vi "Lighting Test Software 4.vi"() -> ()   [LabVIEW 2020]
panel:
  in  "Tab Control":enum32{"Map", "Settings"}(tab)
  in  "Slide":dbl(slide)=0.7342857142857143 scale=0.0..1.0
  in  "Array 3":cluster{"Color Box":u32, "Slide":dbl}[][](array[cluster])=[[{"Color Box"=12303291, "Slide"=10.0}, {"Color Box"=12303291, "Slide"=10.0}, {"Color Box"=12303291, "Slide"=10.0}, {"Color Box"=12303291, "Slide"=10.0}, {"Color Box"=12303291, "Slide"=10.0}, {"Color Box"=12303291, "Slide"=10.0}], [{"Color Box"=12303291, "Slide"=10.0}, {"Color Box"=12303291, "Slide"=10.0}, {"Color Box"=12303291, "Slide"=10.0}, {"Color Box"=12303291, "Slide"=10.0}, {"Color Box"=12303291, "Slide"=10.0}, {"Color Box"=12303291, "Slide"=10.0}], [{"Color Box"=12303291, "Slide"=10.0}, {"Color Box"=12303291, "Slide"=10.0}, {"Color Box"=12303291, "Slide"=10.0}, {"Color Box"=12303291, "Slide"=10.0}, {"Color Box"=12303291, "Slide"=10.0}, {"Color Box"=12303291, "Slide"=10.0}], [{"Color Box"=12303291, "Slide"=10.0}, {"Color Box"=12303291, "Slide"=10.0}, {"Color Box"=12303291, "Slide"=10.0}, {"Color Box"=12303291, "Slide"=10.0}, {"Color Box"=0, "Slide"=0.0}, {"Color Box"=0, "Slide"=0.0}], [{"Color Box"=12303291, "Slide"=10.0}, {"Color Box"=12303291, "Slide"=10.0}, {"Color Box"=0, "Slide"=0.0}, {"Color Box"=12303291, "Slide"=10.0}, {"Color Box"=0, "Slide"=0.0}, {"Color Box"=0, "Slide"=0.0}], [{"Color Box"=0, "Slide"=0.0}, {"Color Box"=0, "Slide"=0.0}, {"Color Box"=12303291, "Slide"=10.0}, {"Color Box"=0, "Slide"=0.0}, {"Color Box"=0, "Slide"=0.0}, {"Color Box"=0, "Slide"=0.0}]] {"Slide" min=0.0 max=10.0 scale=-1.0..11.0 scale format="%_1g"}
  in  "Save Config":bool
  in  "Load Config":bool
  in  "Index":cluster{"Numeric":i32}[][](array[cluster])=[[{"Numeric"=3}, {"Numeric"=9}, {"Numeric"=2}, {"Numeric"=8}, {"Numeric"=19}, {"Numeric"=23}], [{"Numeric"=1}, {"Numeric"=11}, {"Numeric"=0}, {"Numeric"=10}, {"Numeric"=17}, {"Numeric"=21}], [{"Numeric"=5}, {"Numeric"=13}, {"Numeric"=4}, {"Numeric"=14}, {"Numeric"=27}, {"Numeric"=25}], [{"Numeric"=7}, {"Numeric"=15}, {"Numeric"=6}, {"Numeric"=12}, {"Numeric"=26}, {"Numeric"=24}], [{"Numeric"=29}, {"Numeric"=31}, {"Numeric"=-1}, {"Numeric"=18}, {"Numeric"=-1}, {"Numeric"=22}], [{"Numeric"=30}, {"Numeric"=-1}, {"Numeric"=16}, {"Numeric"=-1}, {"Numeric"=-1}, {"Numeric"=-1}]]
  in  "physical channels":refnum<k21>="Dev0/Ao0:15"
  in  "physical channels 2":refnum<k21>="Dev1/Ao0:15"
  out "error out":errorcluster
  out "specific error cleared?":bool
  in  "OK":bool
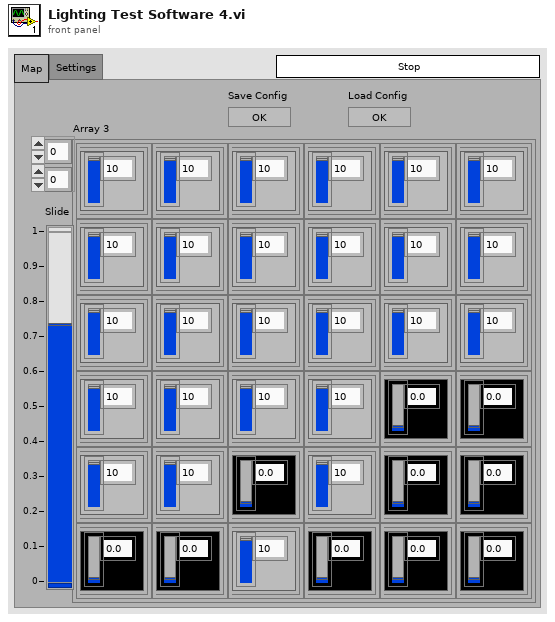
[diagram p1: front panel]
types:
  T1 = enum32{"invalid app kind", "Development System", "Run Time System", "Student Edition", "Embedded LabVIEW", "Evaluation", "Custom"}
  T2 = enum32{"Invalid", "Standard", "Closed", "Hidden", "Minimized", "Maximized"}
  T3 = cluster{"Core":cluster{"Current VI Reference":refnum<vi>, "Close Panel on Exit?":bool}, "Your Boolean data":bool}
  T4 = cluster{"Current VI Reference":refnum<vi>, "Close Panel on Exit?":bool}
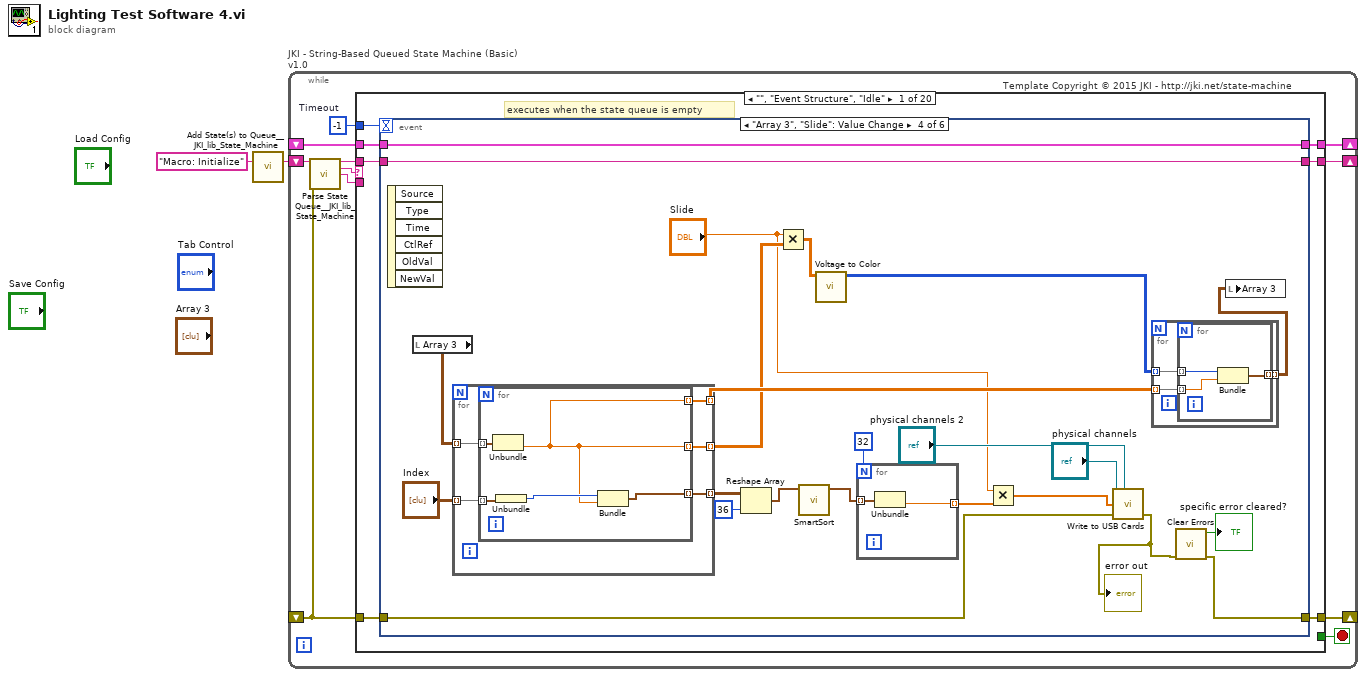
[diagram p0: block diagram]
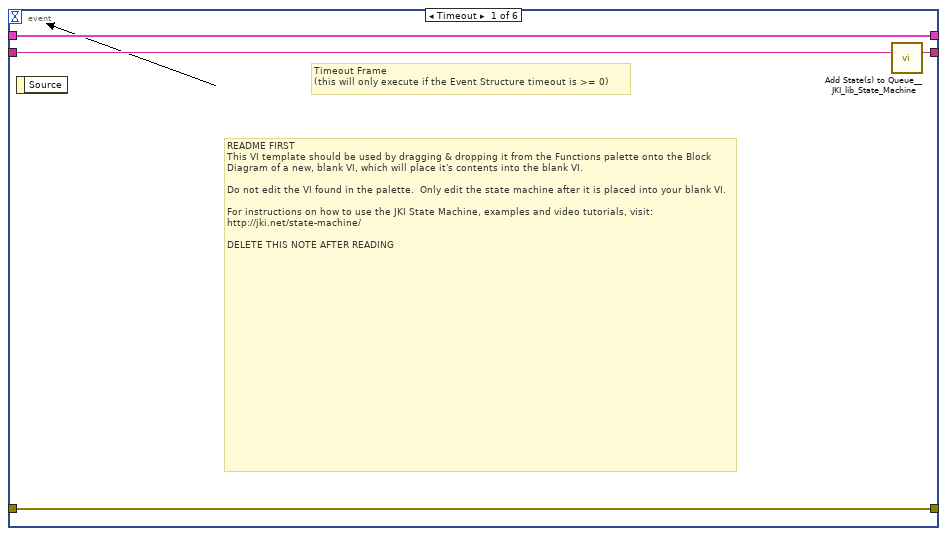
[diagram p2: hidden frame]
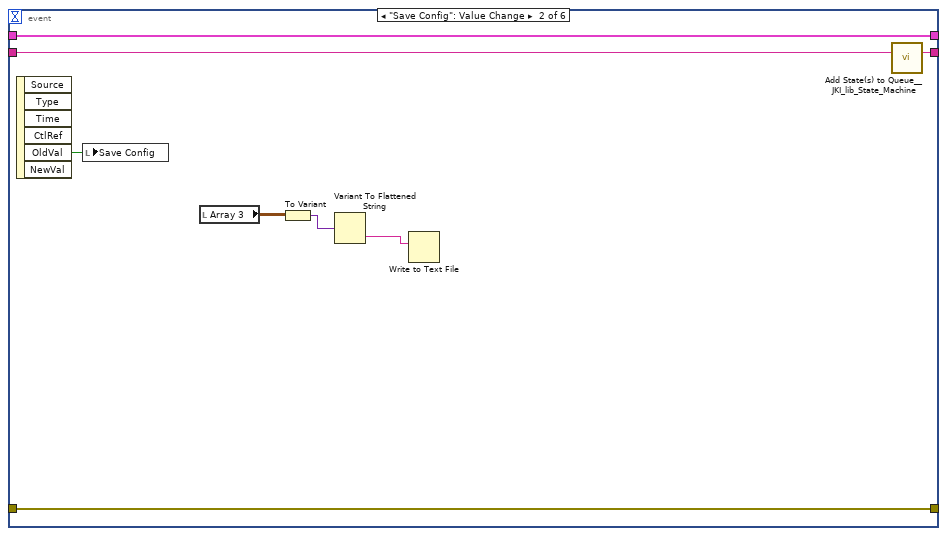
[diagram p3: hidden frame]
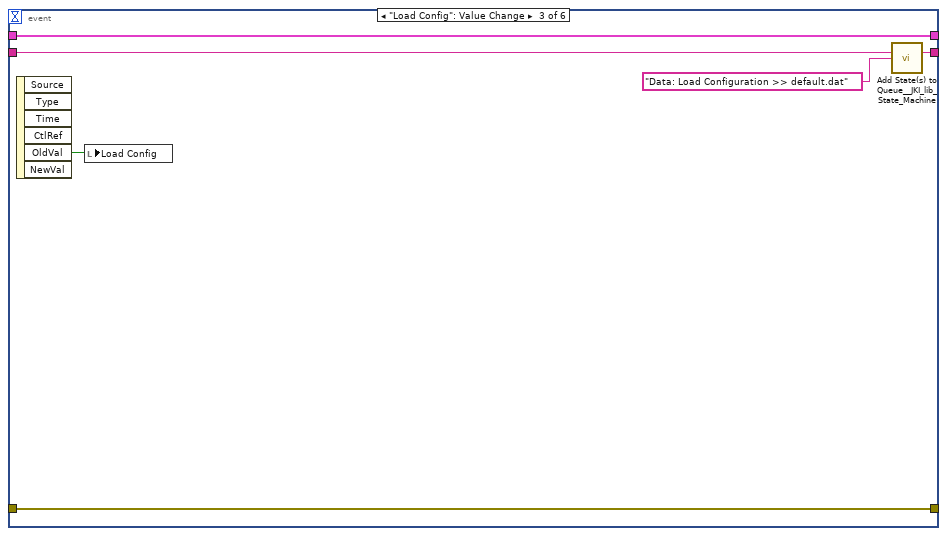
[diagram p4: hidden frame]
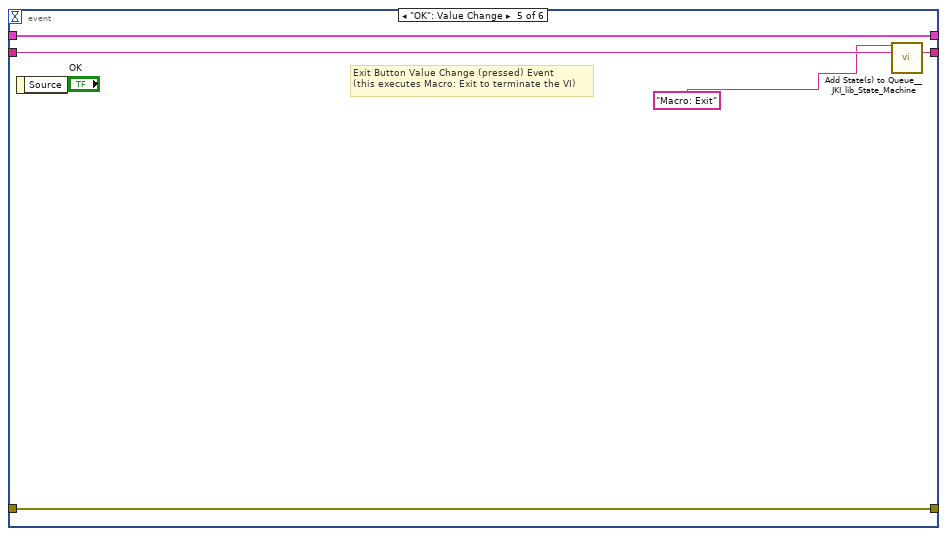
[diagram p5: hidden frame]
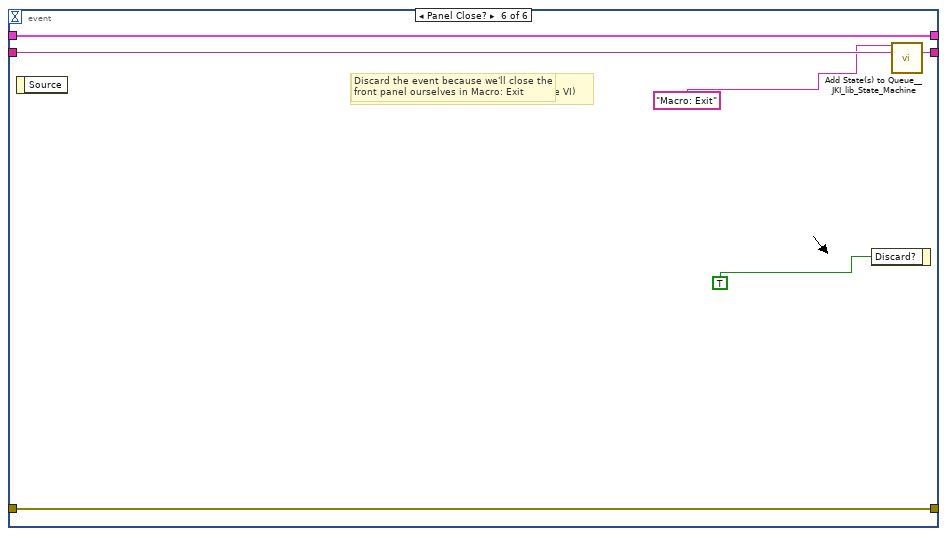
[diagram p6: hidden frame]
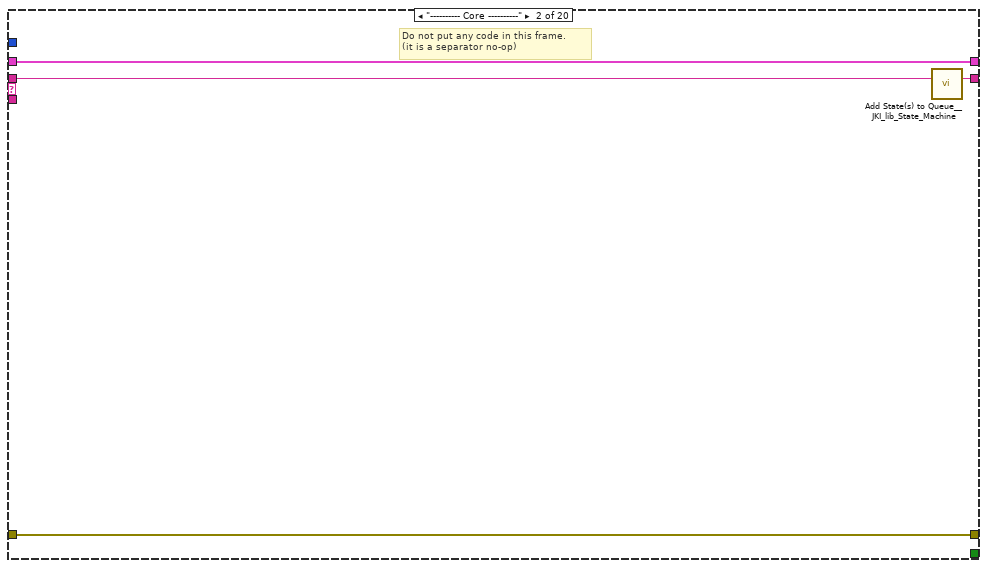
[diagram p7: hidden frame]
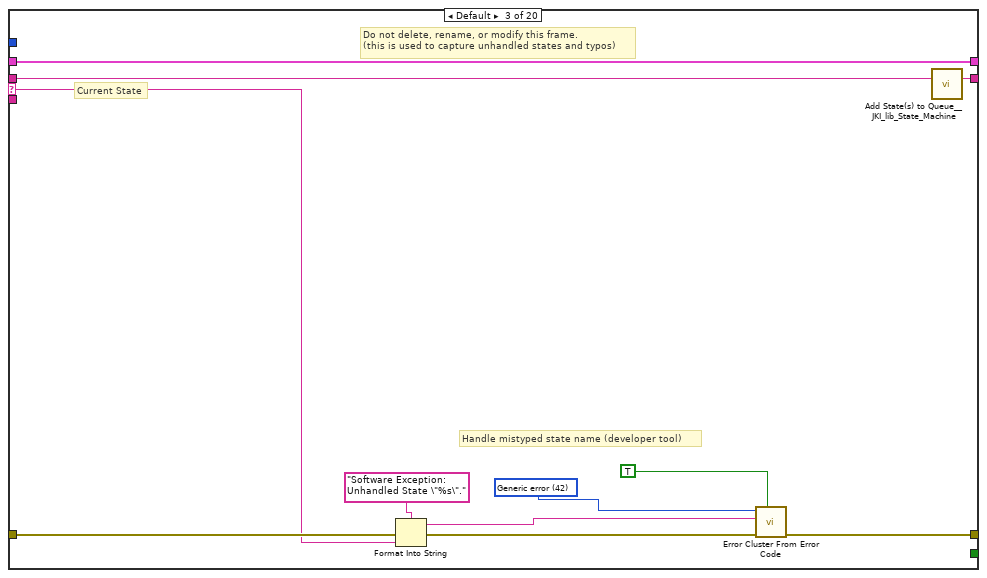
[diagram p8: hidden frame]
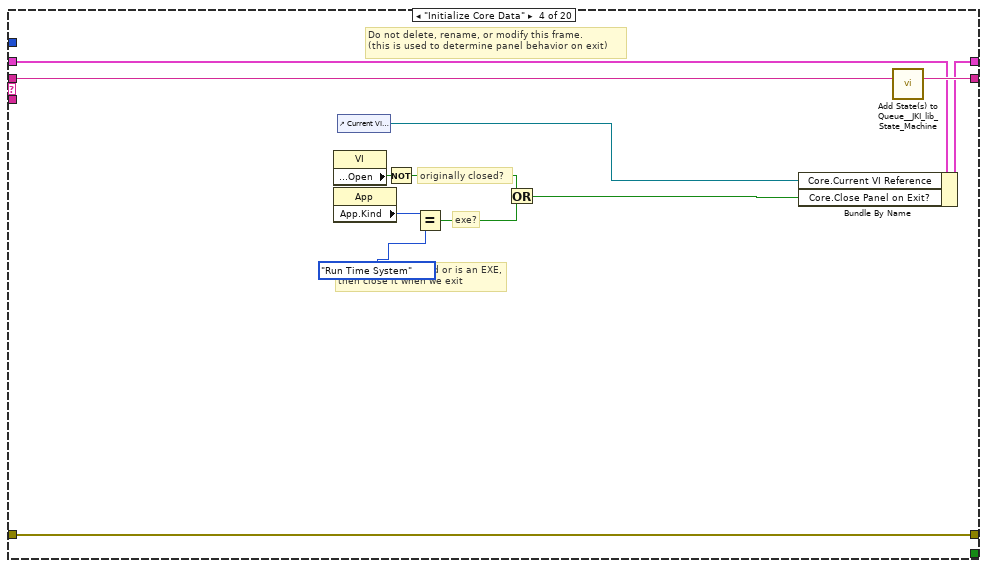
[diagram p9: hidden frame]
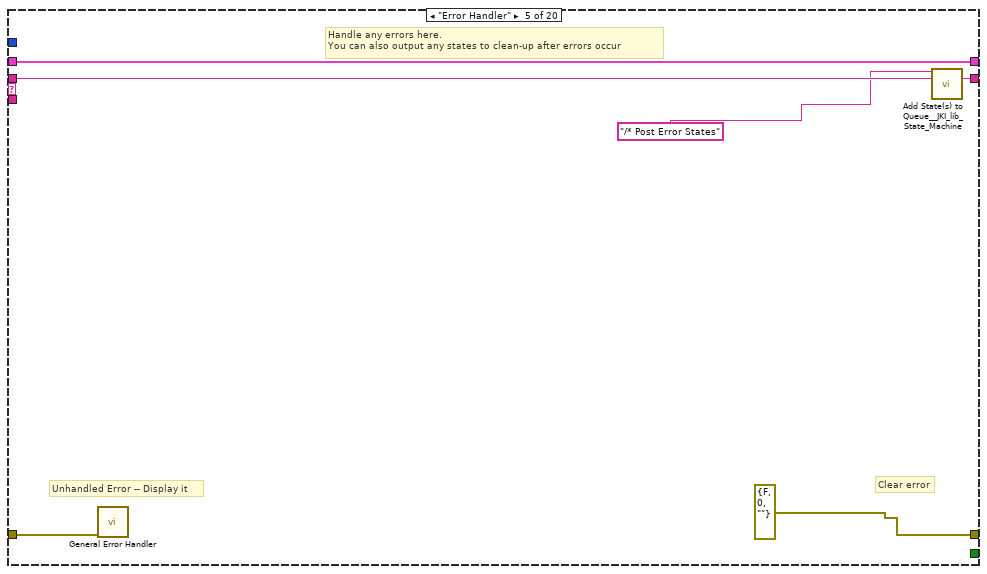
[diagram p10: hidden frame]
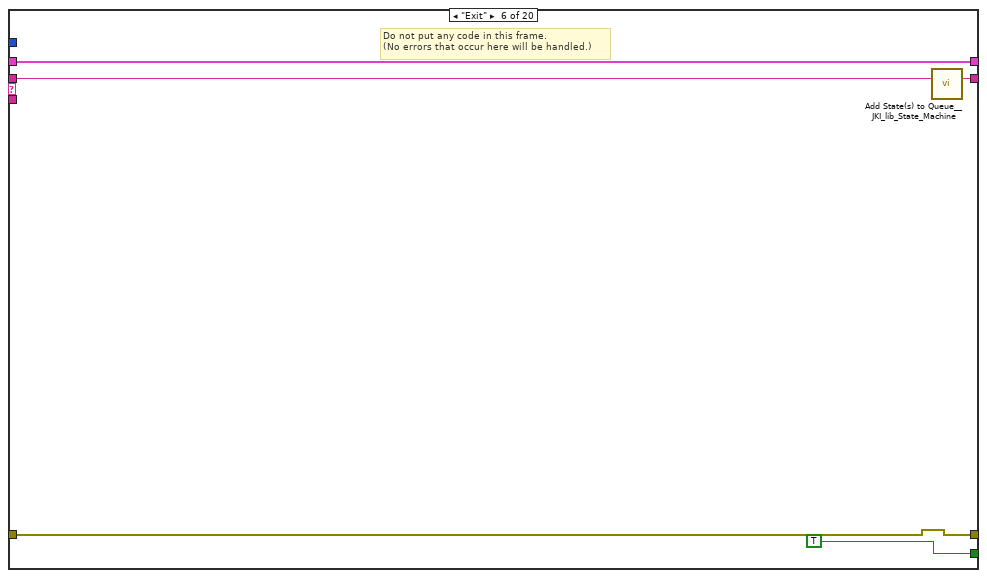
[diagram p11: hidden frame]
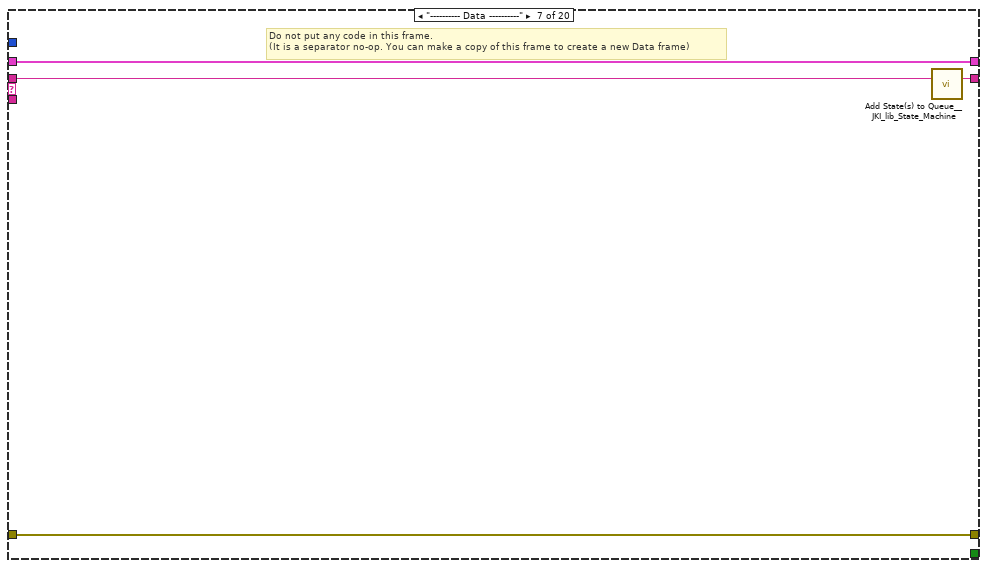
[diagram p12: hidden frame]
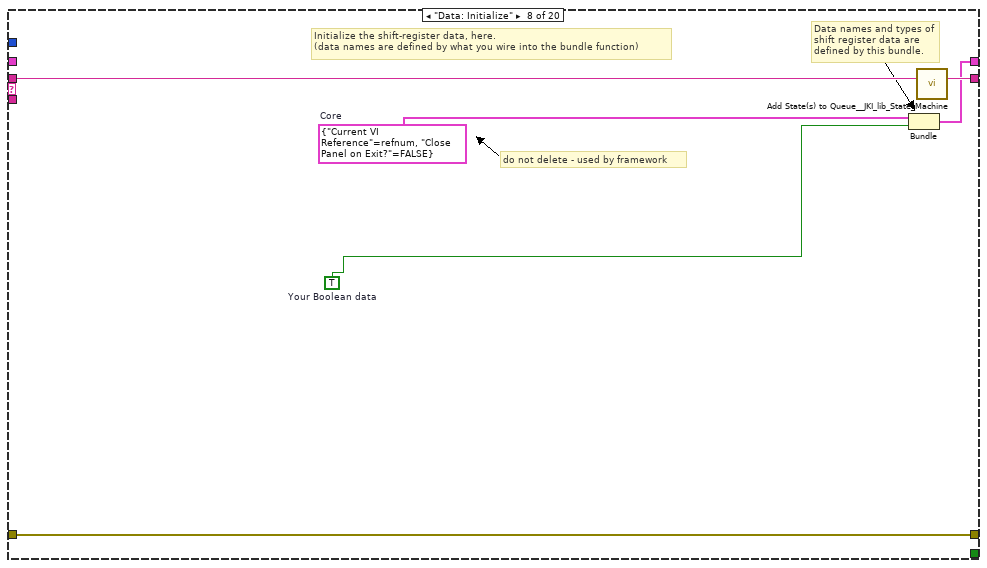
[diagram p13: hidden frame]
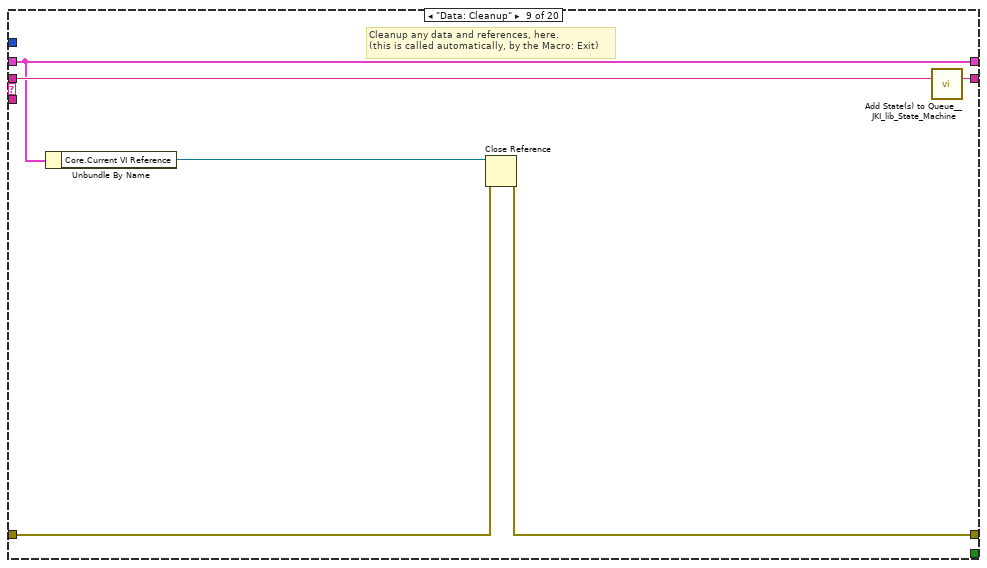
[diagram p14: hidden frame]
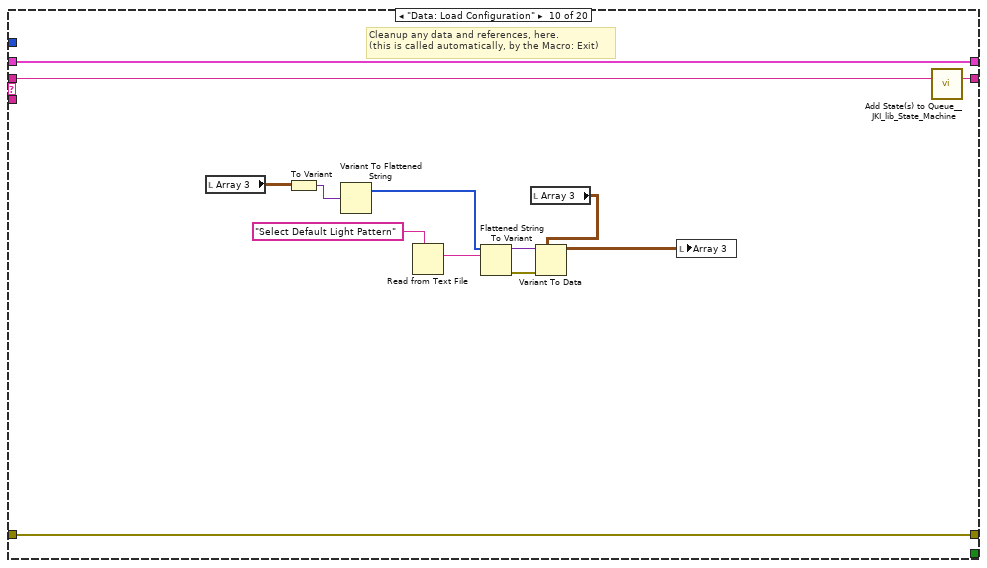
[diagram p15: hidden frame]
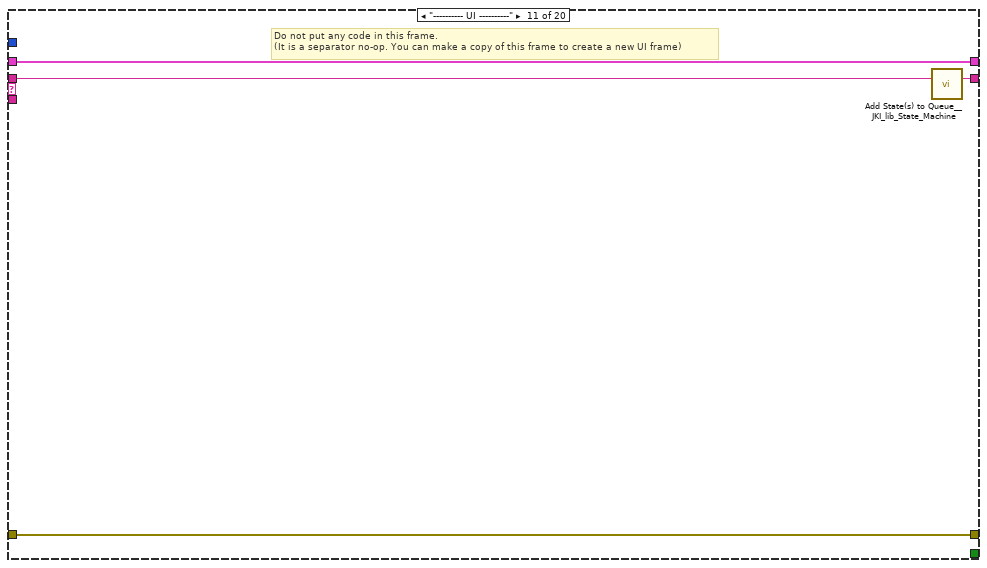
[diagram p16: hidden frame]
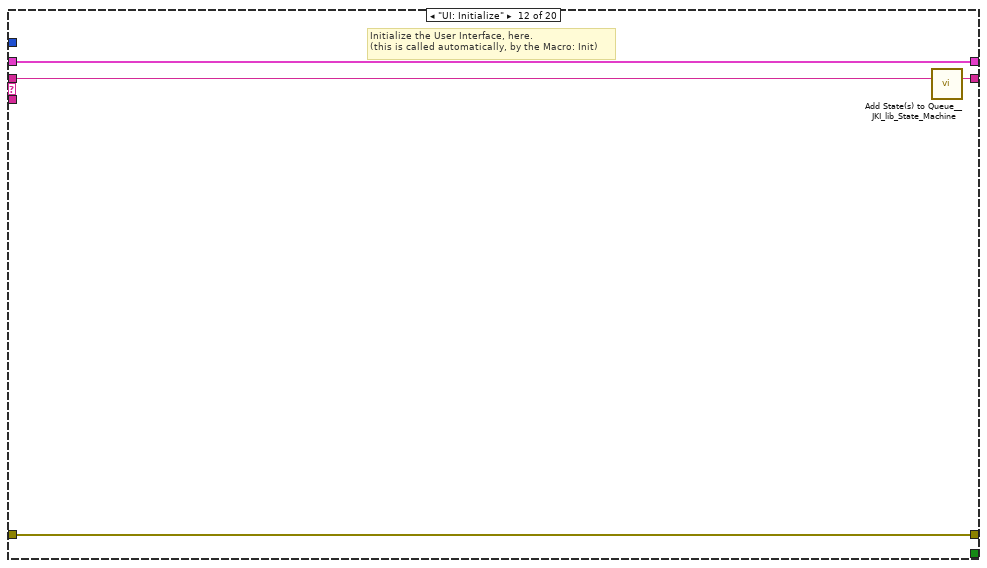
[diagram p17: hidden frame]
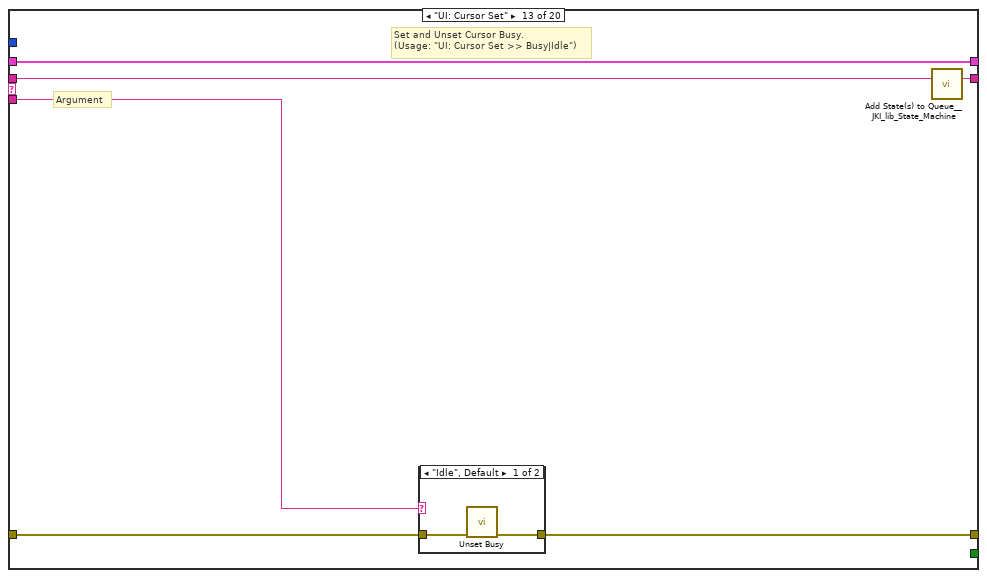
[diagram p18: hidden frame]
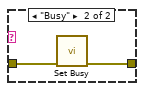
[diagram p19: hidden frame]
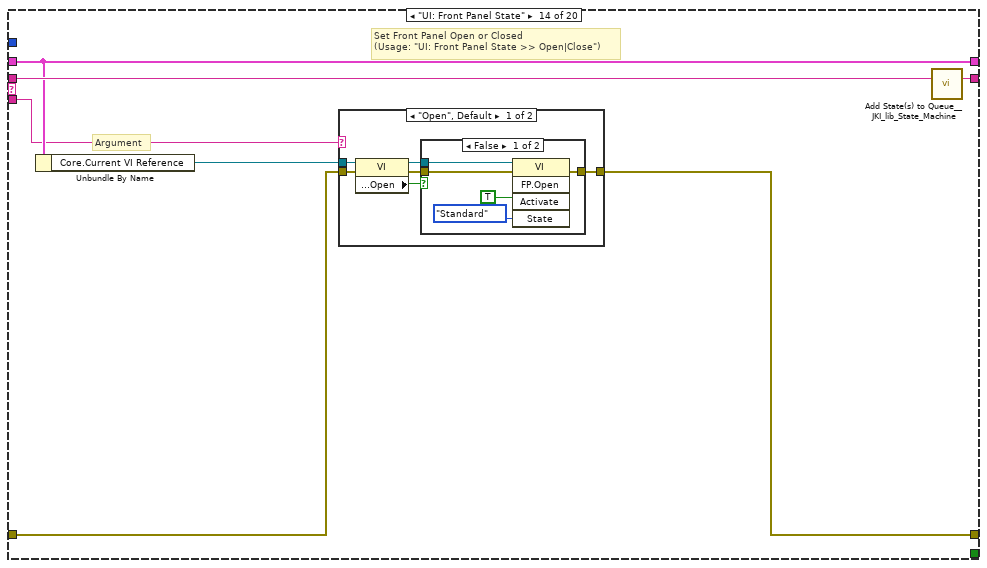
[diagram p20: hidden frame]
diagram:
  n1 = call <vilib>:"Add State(s) to Queue__JKI_lib_State_Machine.vi"("State(s) in (\"\")"="Macro: Initialize") -> ("States Out"=w2:string)  [unwired: 14 in]
  n2 = while "JKI - String-Based Queued State Machine (Basic) v1.0" {
    shift-right: [w6] -> _
    shift-left: _ -> [w5]
    shift-right: [w9] -> _
    shift-left: _ -> [w3]
    shift-right: [w8] -> _
    shift-left: w2 -> [w10]
    stop <- w7 stop-if-true
    w4 = -1  # Timeout
    # "Template Copyright © 2015 JKI - http://jki.net/state-machine"
    n3 = call <vilib>:"Parse State Queue__JKI_lib_State_Machine.vi"("State Queue"=w10, "Error In (no error)"=w3) -> ("Remaining States"=w12:string, "Current State"=w13:string, "Arguments"=w11:string)  [unwired: 11 in]
    n4 = case shown="\"\", \"Event Structure\", \"Idle\"" w13 {
      selector: w13 -> [_ _ w95 _ _ _ _ _ _ _ _ _ _ _ _ _ _ _ _ _]
      tunnel: w12 -> [w20 w94 w99 w117 w123 w128 w132 w138 w144 w157 w161 w165 w171 w182 w208 w213 w223 w227 w231 w235]
      tunnel: w11 -> [_ _ _ _ _ _ _ _ _ _ _ _ w166 w176 _ _ _ _ _ _]
      tunnel: w5 -> [w18 w91 w97 w108 w120 w125 w129 _ w139 w155 w158 w163 w169 w178 w205 w210 w220 w224 w228 w232]
      tunnel: [w17 w92 w101 w114 errorcluster {"status"=FALSE, "code"=0, "source"=""} ("error out") w124 w130 w133 w140 w154 w159 w162 w167 w179 w206 w211 w221 w225 w229 w233] -> w9
      tunnel: w3 -> [w16 w92 w100 w114 w119 w124 w130 w133 w141 w154 w159 w162 w168 w180 w206 w211 w221 w225 w229 w233]
      tunnel: [w19 w93 w98 w116 w122 w127 w131 w137 w143 w156 w160 w164 w170 w181 w207 w212 w222 w226 w230 w234] -> w8
      tunnel: [_ _ _ _ _ TRUE _ _ _ _ _ _ _ _ _ _ _ _ _ _] -> w7
      tunnel: [w15 w91 w97 w115 w120 w125 w129 w136 w139 w155 w158 w163 w169 w178 w205 w210 w220 w224 w228 w232] -> w6
      tunnel: w4 -> [w14 _ _ _ _ _ _ _ _ _ _ _ _ _ _ _ _ _ _ _]
      frame "", "Event Structure", "Idle" {
        # "executes when the state queue is empty"
        n5 = event shown="[3] \"Array 3\", \"Slide\": Value Change" {
          selector: _ -> [_ _ _ _ _ _]
          dyn-events: _ -> [_ _ _ _ _ _]
          timeout: w14 -> [_ _ _ _ _ _]
          tunnel: w20 -> [w24 w32 w38 w60 w84 w90]
          tunnel: [w23 w31 w37 w60 w83 w89] -> w19
          tunnel: w18 -> [w21 w29 w35 w61 w81 w87]
          tunnel: [w22 w30 w36 w46 w82 w88] -> w17
          tunnel: w16 -> [w22 w30 w36 w47 w82 w88]
          tunnel: [w21 w29 w35 w61 w81 w87] -> w15
          event Timeout {
            # "README FIRST\nThis VI template should be used by dragging & dropping it from the Functions palette onto the Block Diagram of a new, blank VI, which will place it's contents into the blank VI.\n\nDo not edit the VI found in the palette.  Only edit the state machine after it is placed into your blank VI.\n\nFor instructions on how to use the JKI State Machine, examples and video tutorials, visit:\nhttp://jki.net/state-machine/\n\nDELETE THIS NOTE AFTER READING"
            # "Timeout Frame\n(this will only execute if the Event Structure timeout is >= 0)"
            n6 = event-data() -> ()  [unwired: 1 in, 1 out]
            n7 = call <vilib>:"Add State(s) to Queue__JKI_lib_State_Machine.vi"("State(s) in (\"\")"=w24) -> ("States Out"=w23:string)  [unwired: 14 in]
          }
          event "Save Config": Value Change {
            n8 = event-data() -> ("OldVal"=w25:bool)  [unwired: 1 in, 5 out]
            n9 = local write "Save Config"(w25) -> ()
            n10 = local read "Array 3"() -> (w28:cluster{"Color Box":u32, "Slide":dbl}[][])
            n11 = To Variant(anything=w28) -> (Variant=w27:variant)
            n12 = Variant To Flattened String(Variant=w27) -> (data string=w26:string)  [unwired: 1 out]
            n13 = Write to Text File(text=w26) -> ()  [unwired: 3 in, 3 out]
            n14 = call <vilib>:"Add State(s) to Queue__JKI_lib_State_Machine.vi"("State(s) in (\"\")"=w32) -> ("States Out"=w31:string)  [unwired: 14 in]
          }
          event "Load Config": Value Change {
            n15 = event-data() -> ("OldVal"=w34:bool)  [unwired: 1 in, 5 out]
            n16 = local write "Load Config"(w34) -> ()
            n17 = call <vilib>:"Add State(s) to Queue__JKI_lib_State_Machine.vi"("State(s) in (\"\")"=w38, "State(s) at Back (\"\")"="Data: Load Configuration >> default.dat") -> ("States Out"=w37:string)  [unwired: 13 in]
          }
          event "Array 3", "Slide": Value Change {
            n18 = event-data() -> ()  [unwired: 1 in, 6 out]
            n19 = local read "Array 3"() -> (w59:cluster{"Color Box":u32, "Slide":dbl}[][])
            n20 = for {
              tunnel: w59 -> [w74] mode=indexing
              tunnel: [w73] -> w43 mode=indexing
              tunnel: [w72] -> w56 mode=indexing
              tunnel: "Index" -> [w71] mode=indexing
              tunnel: [w70] -> w54 mode=indexing
              n21 = for {
                tunnel: w74 -> [w79] mode=indexing
                tunnel: [w76] -> w73 mode=indexing
                tunnel: [w76] -> w72 mode=indexing
                tunnel: w71 -> [w78] mode=indexing
                tunnel: [w75] -> w70 mode=indexing
                n22 = Unbundle(w79) -> ("Slide"=w76:dbl)  [unwired: 1 out]
                n23 = Unbundle(w78) -> ("Numeric"=w77:i32)
                n24 = Bundle("Numeric"=w77, "Slide"=w76) -> (w75:cluster{"Numeric":i32, "Slide":dbl})  [unwired: 1 in]
              }
            }
            n25 = Reshape Array(w54, 36 ("dimension size")) -> (w52:cluster{"Numeric":i32, "Slide":dbl}[])
            n26 = Multiply(x="Slide", y=w43) -> (x*y=w42:dbl[][])
            n27 = call "SmartSort.vi"("Array in"=w52) -> ("Array out"=w51:cluster{"Numeric":i32, "Slide":dbl}[])  [unwired: 10 in]
            n28 = call "Voltage to Color.vi"("Array in"=w42) -> ("Array out"=w57:u32[][])  [unwired: 10 in]
            n29 = for {
              N: 32 -> [_]
              tunnel: w51 -> [w63] mode=indexing
              tunnel: [w62] -> w41 mode=indexing
              n30 = Unbundle(w63) -> ("Slide"=w62:dbl)  [unwired: 1 out]
            }
            n31 = Multiply(x="Slide", y=w41) -> (x*y=w39:dbl[])
            n32 = call "Write to USB Cards.vi"("physical channels"="physical channels", "physical channels 2"="physical channels 2", "Array"=w39, "error in"=w47) -> ("error out"=w44:errorcluster)  [unwired: 5 in]
            "error out" <- w44
            n33 = for {
              tunnel: [w66] -> w58 mode=indexing
              tunnel: w57 -> [w65] mode=indexing
              tunnel: w56 -> [w64] mode=indexing
              n34 = for {
                tunnel: [w69] -> w66 mode=indexing
                tunnel: w65 -> [w68] mode=indexing
                tunnel: w64 -> [w67] mode=indexing
                n35 = Bundle(w68, "Slide"=w67) -> (w69:cluster{u32, "Slide":dbl})  [unwired: 1 in]
              }
            }
            n36 = call <vilib>:"Clear Errors.vi"("error in (no error)"=w44) -> ("error out"=w46:errorcluster, "specific error cleared?"=→"specific error cleared?":bool)  [unwired: 5 in]
            n37 = local write "Array 3"(w58) -> ()
          }
          event "OK": Value Change {
            # "Exit Button Value Change (pressed) Event\n(this executes Macro: Exit to terminate the VI)"
            n38 = event-data() -> ()  [unwired: 1 in, 1 out]
            n39 = call <vilib>:"Add State(s) to Queue__JKI_lib_State_Machine.vi"("State(s) in Front (\"\")"="Macro: Exit", "State(s) in (\"\")"=w84) -> ("States Out"=w83:string)  [unwired: 13 in]
          }
          event Panel Close? {
            # "Discard the event because we'll close the front panel ourselves in Macro: Exit"
            # "Close Panel button (pressed) Event\n(this executes Macro: Exit to terminate the VI)"
            n40 = event-data() -> ()  [unwired: 1 in, 1 out]
            n41 = event-data("Discard?"=TRUE) -> ()  [unwired: 1 in, 1 out]
            n42 = call <vilib>:"Add State(s) to Queue__JKI_lib_State_Machine.vi"("State(s) in Front (\"\")"="Macro: Exit", "State(s) in (\"\")"=w90) -> ("States Out"=w89:string)  [unwired: 13 in]
          }
        }
      }
      frame "---------- Core ----------" {
        # "Do not put any code in this frame.\n(it is a separator no-op)"
        n43 = call <vilib>:"Add State(s) to Queue__JKI_lib_State_Machine.vi"("State(s) in (\"\")"=w94) -> ("States Out"=w93:string)  [unwired: 14 in]
      }
      frame Default {
        w104 = 42 items=["No error", "Argument error", "Memory is full", "Out of zone", "End of file", "File already open", "Generic file I/O error", "File not found", "File permission error", "Disk is full", "Duplicate path", "Too many files open", "System feature not enabled", "Resource file not found", "Cannot add resource", "Resource not found", "Image not found", "Image memory error", "Pen does not exist", "Config type invalid", "Config token not found", "Config parse error", "Config memory error", "Bad external code format", "Bad external code offset", "External code not present", "Null window", "Destroy window error", "Null menu", "Print aborted", "Bad print record", "Print driver error", "Windows error during printing", "Memory error during printing", "Print dialog error", "Generic print error", "Invalid device refnum", "Device not found", "Device parameter error", "Device unit error", "Cannot open device", "Device call aborted", "Generic error", "Cancelled by user", "Object ID too low", "Object ID too high", "Object not in heap", "Unknown heap", "Unknown object (invalid DefProc)", "Unknown object (DefProc not in table)", "Message out of range", "Invalid (null) method", "Unknown message", "Manager call not supported", "Bad address", "Network operation in progress", "Network operation timed out", "Connection is busy", "Network attribute not supported", "Network error", "Address in use", "System out of memory", "Connection aborted", "Connection refused", "Not connected", "Already connected", "Connection closed", "Initialization error (interapplication manager)", "Bad occurrence", "Wait on unbound occurrence handler", "Occurrence queue overflow", "Datalog type conflict", "Unused", "Unrecognized type (interapplication manager)", "Memory corrupt", "Failed to make temporary DLL", "Old CIN version", "Drag socket not found", "Failed to load drop-object", "Failed to register OLE object", "Failed to release OLE object", "Format specifier type mismatch", "Unknown format specifier", "Too few format specifiers", "Too many format specifiers", "Scan failed", "Newer CIN version", "Error converting to variant", "Runtime menu error", "Password tampered", "Variant attribute not found", "Incompatible variant data type", "Event data is not available", "Event Store is not present", "Occurrence is not found", "Event Queue is not created", "Event info is not available", "Refnum passed is NULL", "Error retrieving Class GUID", "Error retrieving CoClass GUID", "Error retrieving TypeLib GUID.", "Bad built application magic bytes.", "Specific driver is different from the specific driver associated with the Logical Name.", "There is no session opened to the class driver.", "Max Error", "MAX - Error with config objects", "MAX - Error loading configuration", "MAX - Group not supported"]
        # "Current State"
        # "Do not delete, rename, or modify this frame.\n(this is used to capture unhandled states and typos)"
        # "Handle mistyped state name (developer tool)"
        n44 = Format Into String(format string="Software Exception: Unhandled State \"%s\"." ("message"), error in=w100, w95) -> (resulting string=w103:string, error out=w102:errorcluster)  [unwired: 1 in]
        n45 = call <vilib>:"Error Cluster From Error Code.vi"("show call chain? (False)"=TRUE, "error in (no error)"=w102, "error message (\"\")"=w103, "error code (0)"=w104) -> ("error out"=w101:errorcluster)  [unwired: 5 in]
        n46 = call <vilib>:"Add State(s) to Queue__JKI_lib_State_Machine.vi"("State(s) in (\"\")"=w99) -> ("States Out"=w98:string)  [unwired: 14 in]
      }
      frame "Initialize Core Data" {
        # "Do not delete, rename, or modify this frame.\n(this is used to determine panel behavior on exit)"
        # "originally closed?"
        # "exe?"
        # "If panel starts closed or is an EXE, then close it when we exit"
        n47 = property class="VI"() -> ("Front Panel.Open"=w113:bool)  [unwired: 2 in, 2 out]
        n48 = property class="App"() -> ("App.Kind"=w112:T1)  [unwired: 2 in, 2 out]
        n49 = control-ref of="Current VI Reference"() -> (w106:refnum<vi>)
        n50 = Not(x=w113) -> (.not. x?=w110:bool)
        n51 = Equal?(x=w112, y=T1."Run Time System" ("Application:Kind")) -> (x = y?=w109:bool)
        n52 = Or(x=w110, y=w109) -> (x .or. y?=w107:bool)
        n53 = Bundle By Name(cluster=w108, "Core.Current VI Reference"=w106, "Core.Close Panel on Exit?"=w107) -> (w115:T3)
        n54 = call <vilib>:"Add State(s) to Queue__JKI_lib_State_Machine.vi"("State(s) in (\"\")"=w117) -> ("States Out"=w116:string)  [unwired: 14 in]
      }
      frame "Error Handler" {
        # "Unhandled Error -- Display it"
        # "Handle any errors here.\nYou can also output any states to clean-up after errors occur"
        # "Clear error"
        n55 = call <vilib>:"General Error Handler.vi"("error in (no error)"=w119) -> ()  [unwired: 10 in, 5 out]
        n56 = call <vilib>:"Add State(s) to Queue__JKI_lib_State_Machine.vi"("State(s) in Front (\"\")"="/* Post Error States", "State(s) in (\"\")"=w123) -> ("States Out"=w122:string)  [unwired: 13 in]
      }
      frame "Exit" {
        # "Do not put any code in this frame.\n(No errors that occur here will be handled.)"
        n57 = call <vilib>:"Add State(s) to Queue__JKI_lib_State_Machine.vi"("State(s) in (\"\")"=w128) -> ("States Out"=w127:string)  [unwired: 14 in]
      }
      frame "---------- Data ----------" {
        # "Do not put any code in this frame.\n(It is a separator no-op. You can make a copy of this frame to create a new Data frame)"
        n58 = call <vilib>:"Add State(s) to Queue__JKI_lib_State_Machine.vi"("State(s) in (\"\")"=w132) -> ("States Out"=w131:string)  [unwired: 14 in]
      }
      frame "Data: Initialize" {
        w134 = T4 {"Current VI Reference"=refnum, "Close Panel on Exit?"=FALSE}  # Core
        w135 = TRUE  # Your Boolean data
        # "do not delete - used by framework"
        # "Data names and types of shift register data are defined by this bundle."
        # "Initialize the shift-register data, here.\n(data names are defined by what you wire into the bundle function)"
        n59 = Bundle("Core"=w134, "Your Boolean data"=w135) -> (w136:T3)  [unwired: 1 in]
        n60 = call <vilib>:"Add State(s) to Queue__JKI_lib_State_Machine.vi"("State(s) in (\"\")"=w138) -> ("States Out"=w137:string)  [unwired: 14 in]
      }
      frame "Data: Cleanup" {
        # "Cleanup any data and references, here.\n(this is called automatically, by the Macro: Exit)"
        n61 = Unbundle By Name(w139) -> ("Core.Current VI Reference"=w142:refnum<vi>)
        n62 = Close Reference(reference=w142, error in (no error)=w141) -> (error out=w140:errorcluster)
        n63 = call <vilib>:"Add State(s) to Queue__JKI_lib_State_Machine.vi"("State(s) in (\"\")"=w144) -> ("States Out"=w143:string)  [unwired: 14 in]
      }
      frame "Data: Load Configuration" {
        # "Cleanup any data and references, here.\n(this is called automatically, by the Macro: Exit)"
        n64 = local read "Array 3"() -> (w153:cluster{"Color Box":u32, "Slide":dbl}[][])
        n65 = To Variant(anything=w153) -> (Variant=w148:variant)
        n66 = Variant To Flattened String(Variant=w148) -> (1:w151:i16[])  [unwired: 1 out]
        n67 = Read from Text File(prompt (Open existing file)="Select Default Light Pattern") -> (text=w152:string)  [unwired: 3 in, 3 out]
        n68 = Flattened String To Variant(6:w152, 7:w151) -> (0:w150:errorcluster, 3:w149:variant)  [unwired: 1 in]
        n69 = local read "Array 3"() -> (w146:cluster{"Color Box":u32, "Slide":dbl}[][])
        n70 = Variant To Data(error in=w150, type=w146, Variant=w149) -> (data=w147:cluster{"Color Box":u32, "Slide":dbl}[][])  [unwired: 1 out]
        n71 = local write "Array 3"(w147) -> ()
        n72 = call <vilib>:"Add State(s) to Queue__JKI_lib_State_Machine.vi"("State(s) in (\"\")"=w157) -> ("States Out"=w156:string)  [unwired: 14 in]
      }
      frame "---------- UI ----------" {
        # "Do not put any code in this frame.\n(It is a separator no-op. You can make a copy of this frame to create a new UI frame)"
        n73 = call <vilib>:"Add State(s) to Queue__JKI_lib_State_Machine.vi"("State(s) in (\"\")"=w161) -> ("States Out"=w160:string)  [unwired: 14 in]
      }
      frame "UI: Initialize" {
        # "Initialize the User Interface, here.\n(this is called automatically, by the Macro: Init)"
        n74 = call <vilib>:"Add State(s) to Queue__JKI_lib_State_Machine.vi"("State(s) in (\"\")"=w165) -> ("States Out"=w164:string)  [unwired: 14 in]
      }
      frame "UI: Cursor Set" {
        # "Argument"
        # "Set and Unset Cursor Busy.\n(Usage: \"UI: Cursor Set >> Busy|Idle\")"
        n75 = case shown="\"Idle\", Default" w166 {
          tunnel: w168 -> [w173 w175]
          tunnel: [w172 w174] -> w167
          frame "Idle", Default {
            n76 = call <vilib>:"Unset Busy.vi"("error in (no error)"=w173) -> ("error out"=w172:errorcluster)  [unwired: 10 in]
          }
          frame "Busy" {
            n77 = call <vilib>:"Set Busy.vi"("error in (no error)"=w175) -> ("error out"=w174:errorcluster)  [unwired: 9 in, 1 out]
          }
        }
        n78 = call <vilib>:"Add State(s) to Queue__JKI_lib_State_Machine.vi"("State(s) in (\"\")"=w171) -> ("States Out"=w170:string)  [unwired: 14 in]
      }
      frame "UI: Front Panel State" {
        # "Argument"
        # "Set Front Panel Open or Closed\n(Usage: \"UI: Front Panel State >> Open|Close\")"
        n79 = Unbundle By Name(w178) -> ("Core.Current VI Reference"=w177:refnum<vi>)
        n80 = case shown="\"Open\", Default" w176 {
          tunnel: w180 -> [w186 w199]
          tunnel: [w188 w200] -> w179
          tunnel: w177 -> [w187 w197]
          frame "Open", Default {
            n81 = property class="VI"(reference=w187, error in=w186) -> (reference out=w184:refnum<vi>, error out=w185:errorcluster, "Front Panel.Open"=w183:bool)
            n82 = case shown="False" w183 {
              tunnel: [w191 w194] -> w188
              tunnel: w185 -> [w190 w194]
              tunnel: w184 -> [w189 _]
              frame False {
                n83 = invoke class="VI" method="FP.Open"(reference=w189, error in=w190, "Activate"=TRUE, "State"=T2."Standard") -> (error out=w191:errorcluster)  [unwired: 1 in, 4 out]
              }
              frame True {
              }
            }
          }
          frame "Close" {
            n84 = property class="VI"(reference=w197, error in=w199) -> (reference out=w196:refnum<vi>, error out=w198:errorcluster, "Front Panel.Open"=w195:bool)
            n85 = case shown="True" w195 {
              tunnel: [w201 w204] -> w200
              tunnel: w198 -> [w201 w203]
              tunnel: w196 -> [_ w202]
              frame False {
              }
              frame True {
                n86 = invoke class="VI" method="FP.Close"(reference=w202, error in=w203) -> (error out=w204:errorcluster)  [unwired: 1 in, 2 out]
              }
            }
          }
        }
        n87 = call <vilib>:"Add State(s) to Queue__JKI_lib_State_Machine.vi"("State(s) in (\"\")"=w182) -> ("States Out"=w181:string)  [unwired: 14 in]
      }
      frame "---------- Macro ----------" {
        # "Do not put any code in this frame.\n(It is a separator no-op. You can make a copy of this frame to create a new Macro frame)"
        n88 = call <vilib>:"Add State(s) to Queue__JKI_lib_State_Machine.vi"("State(s) in (\"\")"=w208) -> ("States Out"=w207:string)  [unwired: 14 in]
      }
      frame "Macro: Initialize" {
        w209 = "Data: Initialize\nInitialize Core Data\nUI: Initialize\nUI: Front Panel State >> Open"  # Data: Initialize Initialize Core Data UI: Initialize UI: Front Panel State >> Open
        # "Initialization Macro\n(This is called once, when the VI starts)"
        n89 = call <vilib>:"Add State(s) to Queue__JKI_lib_State_Machine.vi"("State(s) in Front (\"\")"=w209, "State(s) in (\"\")"=w213) -> ("States Out"=w212:string)  [unwired: 13 in]
      }
      frame "Macro: Exit" {
        # "Exit Macro\n(This is called once, when the VI exits)"
        n90 = Unbundle By Name(w220) -> ("Core.Close Panel on Exit?"=w219:bool)
        n91 = Select(t="UI: Front Panel State >> Close", s=w219, f="") -> (s? t:f=w216:string)
        n92 = call <vilib>:"Add State(s) to Queue__JKI_lib_State_Machine.vi"("State(s) in (\"\")"=w216, "State(s) at Back (\"\")"="Data: Cleanup\nExit") -> ("States Out"=w214:string)  [unwired: 13 in]
        n93 = call <vilib>:"Add State(s) to Queue__JKI_lib_State_Machine.vi"("State(s) in Front (\"\")"=w214, "State(s) in (\"\")"=w223) -> ("States Out"=w222:string)  [unwired: 13 in]
      }
      frame "---------- New Category ----------" {
        # "Template Separator\n(You can make a copy of, or modify, this frame)"
        n94 = call <vilib>:"Add State(s) to Queue__JKI_lib_State_Machine.vi"("State(s) in (\"\")"=w227) -> ("States Out"=w226:string)  [unwired: 14 in]
      }
      frame "New Category: 1" {
        # "Your code here.\n(You can make a copy of, or modify, this frame)"
        n95 = call <vilib>:"Add State(s) to Queue__JKI_lib_State_Machine.vi"("State(s) in (\"\")"=w231) -> ("States Out"=w230:string)  [unwired: 14 in]
      }
      frame "New Category: 2" {
        # "Your code here.\n(You can make a copy of, or modify, this frame)"
        n96 = call <vilib>:"Add State(s) to Queue__JKI_lib_State_Machine.vi"("State(s) in (\"\")"=w235) -> ("States Out"=w234:string)  [unwired: 14 in]
      }
    }
  }
